vi "Backup.vi"() -> ()   [LabVIEW 2013]
uses:
  GUI_Template/GUI_master/tcp_new_data_event.ctl
  GUI_Template/GUI_master/tcp new data cluster.ctl
  <vilib>/vision/NI_Vision_Development_Module.lvlib
panel:
  out "MagSpec Lineout":cluster{"energy":dbl[], "counts":dbl[]}[](graph)=[{"energy"=array[427 elements], "counts"=[480.0, 481.0, 470.0, 482.0, 477.0, 480.0, 479.0, 479.0, 480.0, 485.0, 481.0, 484.0, 483.0, 482.0, 483.0, 477.0, 477.0, 475.0, 479.0, 479.0, 485.0, 477.0, 480.0, 478.0, 475.0, 485.0, 477.0, 485.0, 472.0, 479.0, 479.0, 472.0, 480.0, 481.0, 482.0, 481.0, 479.0, 477.0, 481.0, 486.0, 477.0, 477.0, 482.0, 481.0, 493.0, 474.0, 491.0, 486.0, 494.0, 488.0, 508.0, 495.0, 494.0, 499.0, 511.0, 500.0, 503.0, 501.0, 496.0, 499.0, 497.0, 500.0, 496.0, 503.0, 501.0, 504.0, 493.0, 492.0, 492.0, 492.0, 500.0, 494.0, 506.0, 494.0, 498.0, 492.0, 498.0, 503.0, 507.0, 498.0, 507.0, 504.0, 506.0, 504.0, 505.0, 503.0, 509.0, 501.0, 502.0, 500.0, 500.0, 496.0, 490.0, 491.0, 483.0, 490.0, 484.0, 469.0, 473.0, 469.0, 469.0, 469.0, 456.0, 465.0, 456.0, 458.0, 451.0, 445.0, 450.0, 443.0, 454.0, 438.0, 434.0, 440.0, 442.0, 450.0, 447.0, 447.0, 450.0, 446.0, 444.0, 446.0, 445.0, 433.0, 449.0, 444.0, 443.0, 441.0, 440.0, 436.0, 444.0, 440.0, 439.0, 435.0, 438.0, 430.0, 435.0, 432.0, 428.0, 433.0, 432.0, 430.0, 434.0, 428.0, 441.0, 426.0, 429.0, 427.0, 425.0, 423.0, 424.0, 419.0, 423.0, 428.0, 423.0, 423.0, 421.0, 423.0, 425.0, 425.0, 419.0, 426.0, 430.0, 429.0, 423.0, 423.0, 422.0, 421.0, 427.0, 426.0, 427.0, 420.0, 416.0, 428.0, 422.0, 420.0, 420.0, 422.0, 428.0, 423.0, 433.0, 417.0, 431.0, 419.0, 428.0, 427.0, 423.0, 417.0, 427.0, 419.0, 422.0, 421.0, 427.0, 420.0, 426.0, 419.0, 430.0, 422.0, 425.0, 426.0, 426.0, 422.0, 434.0, 427.0, 425.0, 430.0, 437.0, 434.0, 432.0, 441.0, 434.0, 435.0, 433.0, 434.0, 439.0, 434.0, 441.0, 436.0, 442.0, 440.0, 443.0, 446.0, 449.0, 441.0, 444.0, 441.0, 448.0, 455.0, 462.0, 450.0, 452.0, 452.0, 465.0, 463.0, 469.0, 466.0, 464.0, 462.0, 476.0, 460.0, 462.0, 475.0, 472.0, 473.0, 477.0, 471.0, 485.0, 474.0, 491.0, 482.0, 485.0, 492.0, 494.0, 498.0, 503.0, 491.0, 500.0, 501.0, 516.0, 500.0, 507.0, 515.0, 523.0, 517.0, 519.0, 525.0, 523.0, 521.0, 524.0, 528.0, 537.0, 533.0, 533.0, 542.0, 548.0, 538.0, 551.0, 563.0, 557.0, 565.0, 559.0, 570.0, 565.0, 580.0, 580.0, 578.0, 586.0, 591.0, 596.0, 605.0, 609.0, 607.0, 614.0, 620.0, 621.0, 628.0, 634.0, 642.0, 654.0, 646.0, 661.0, 654.0, 667.0, 676.0, 681.0, 683.0, 689.0, 703.0, 706.0, 725.0, 719.0, 744.0, 747.0, 757.0, 763.0, 773.0, 794.0, 795.0, 808.0, 821.0, 835.0, 838.0, 853.0, 861.0, 869.0, 886.0, 911.0, 903.0, 902.0, 916.0, 935.0, 925.0, 941.0, 959.0, 967.0, 966.0, 984.0, 976.0, 987.0, 1012.0, 1017.0, 1022.0, 1033.0, 1050.0, 1054.0, 1058.0, 1058.0, 1075.0, 1086.0, 1087.0, 1103.0, 1101.0, 1110.0, 1112.0, 1126.0, 1138.0, 1134.0, 1144.0, 1157.0, 1154.0, 1160.0, 1163.0, 1169.0, 1171.0, 1182.0, 1188.0, 1205.0, 1211.0, 1227.0, 1220.0, 1233.0, 1235.0, 1238.0, 1243.0, 1277.0, 1277.0, 1288.0, 1312.0, 1332.0, 1352.0, 1362.0, 1370.0, 1389.0, 1395.0, 1421.0, 1435.0, 1454.0, 1462.0, 1485.0, 1494.0, 1503.0, 1520.0, 1543.0, 1547.0, 1566.0, 1577.0, 1593.0, 1602.0, 1618.0, 1614.0, 1617.0, 1635.0, 1639.0, 1657.0, 1672.0, 1671.0, 1687.0, 1690.0, 1698.0, 1721.0, 1734.0, 1738.0, 1760.0, 1753.0, 1769.0, 1785.0, 1780.0, 1802.0, 1812.0, 1813.0, 1836.0, 1833.0, 1846.0, 1851.0, 1867.0, 1867.0, 1877.0]}, {"energy"=array[422 elements], "counts"=[1920.0, 1960.0, 1978.0, 1986.0, 2002.0, 2034.0, 2037.0, 2038.0, 2026.0, 2017.0, 2022.0, 2022.0, 2018.0, 2053.0, 2099.0, 2108.0, 2128.0, 2125.0, 2140.0, 2134.0, 2113.0, 2043.0, 1933.0, 1867.0, 1774.0, 1644.0, 1490.0, 1401.0, 1400.0, 1387.0, 1372.0, 1371.0, 1376.0, 1391.0, 1450.0, 1556.0, 1656.0, 1756.0, 1813.0, 1848.0, 1821.0, 1828.0, 1878.0, 1905.0, 1924.0, 1942.0, 1951.0, 1931.0, 1918.0, 1911.0, 1908.0, 1907.0, 1901.0, 1880.0, 1802.0, 1645.0, 1677.0, 1822.0, 1845.0, 1854.0, 1852.0, 1859.0, 1860.0, 1856.0, 1847.0, 1859.0, 1851.0, 1834.0, 1846.0, 1825.0, 1796.0, 1816.0, 1790.0, 1790.0, 1768.0, 1765.0, 1739.0, 1738.0, 1724.0, 1712.0, 1701.0, 1668.0, 1651.0, 1623.0, 1523.0, 1495.0, 1579.0, 1586.0, 1585.0, 1569.0, 1553.0, 1538.0, 1524.0, 1521.0, 1493.0, 1498.0, 1482.0, 1474.0, 1449.0, 1435.0, 1422.0, 1435.0, 1428.0, 1421.0, 1409.0, 1409.0, 1397.0, 1393.0, 1373.0, 1361.0, 1348.0, 1349.0, 1318.0, 1284.0, 1227.0, 1271.0, 1281.0, 1285.0, 1262.0, 1274.0, 1262.0, 1266.0, 1247.0, 1241.0, 1229.0, 1227.0, 1205.0, 1207.0, 1183.0, 1171.0, 1175.0, 1171.0, 1168.0, 1166.0, 1147.0, 1155.0, 1133.0, 1135.0, 1132.0, 1120.0, 1106.0, 1091.0, 1080.0, 1031.0, 1029.0, 1065.0, 1054.0, 1067.0, 1054.0, 1042.0, 1039.0, 1041.0, 1034.0, 1021.0, 1020.0, 999.0, 989.0, 983.0, 972.0, 978.0, 965.0, 960.0, 946.0, 951.0, 942.0, 938.0, 924.0, 917.0, 906.0, 908.0, 902.0, 881.0, 857.0, 842.0, 848.0, 858.0, 853.0, 855.0, 866.0, 849.0, 848.0, 837.0, 826.0, 812.0, 778.0, 726.0, 696.0, 683.0, 698.0, 694.0, 683.0, 681.0, 697.0, 698.0, 672.0, 668.0, 660.0, 667.0, 672.0, 686.0, 695.0, 701.0, 685.0, 685.0, 735.0, 763.0, 773.0, 792.0, 785.0, 791.0, 786.0, 792.0, 782.0, 780.0, 771.0, 777.0, 774.0, 761.0, 762.0, 769.0, 770.0, 767.0, 774.0, 765.0, 766.0, 761.0, 759.0, 762.0, 753.0, 752.0, 745.0, 739.0, 716.0, 710.0, 728.0, 749.0, 745.0, 747.0, 732.0, 751.0, 739.0, 744.0, 729.0, 734.0, 727.0, 723.0, 721.0, 719.0, 713.0, 716.0, 715.0, 716.0, 703.0, 721.0, 704.0, 708.0, 698.0, 695.0, 688.0, 692.0, 674.0, 678.0, 632.0, 646.0, 659.0, 679.0, 676.0, 674.0, 669.0, 664.0, 659.0, 668.0, 654.0, 650.0, 645.0, 650.0, 640.0, 635.0, 630.0, 635.0, 630.0, 637.0, 622.0, 621.0, 626.0, 614.0, 606.0, 614.0, 599.0, 597.0, 589.0, 580.0, 564.0, 575.0, 584.0, 590.0, 584.0, 585.0, 579.0, 582.0, 578.0, 571.0, 573.0, 574.0, 560.0, 559.0, 553.0, 547.0, 545.0, 554.0, 544.0, 553.0, 537.0, 540.0, 536.0, 539.0, 531.0, 525.0, 527.0, 522.0, 511.0, 497.0, 482.0, 503.0, 507.0, 515.0, 501.0, 503.0, 503.0, 502.0, 492.0, 485.0, 485.0, 483.0, 481.0, 479.0, 475.0, 460.0, 467.0, 462.0, 461.0, 466.0, 460.0, 463.0, 452.0, 448.0, 453.0, 446.0, 438.0, 423.0, 407.0, 366.0, 390.0, 423.0, 422.0, 433.0, 428.0, 418.0, 409.0, 419.0, 412.0, 418.0, 410.0, 407.0, 401.0, 397.0, 393.0, 404.0, 395.0, 390.0, 388.0, 395.0, 387.0, 386.0, 383.0, 385.0, 372.0, 370.0, 361.0, 360.0, 338.0, 338.0, 352.0, 364.0, 358.0, 351.0, 350.0, 348.0, 344.0, 346.0, 344.0, 343.0, 335.0, 340.0, 326.0, 327.0, 327.0, 328.0, 330.0, 328.0, 326.0, 316.0, 317.0, 320.0, 312.0, 325.0, 305.0, 306.0, 301.0, 287.0, 271.0, 290.0, 296.0, 294.0, 290.0, 293.0, 295.0, 284.0, 286.0, 283.0, 279.0, 281.0]}, {"energy"=array[479 elements], "counts"=array[479 elements]}]
  in  "confg cluster Cam2":T1={"position"=19.22, "field of view"=279.27, "Analysis ROI"=[23, 41, 501, 146]}
  in  "confg cluster Cam1":T1={"position"=142.68, "field of view"=174.3, "Analysis ROI"=[20, 85, 441, 119]}
  in  "confg cluster Cam0":T1={"position"=45.72, "field of view"=106.18, "Analysis ROI"=[50, 122, 476, 184]}
  out "image::5":T2(plugin-control) caption="MagSpec2"
  out "MagSpec2":u8[][](graph)
  out "error out":errorcluster
  out "image::4":T2(plugin-control) caption="MagSpec1"
  out "MagSpec1":u8[][](graph)
  in  "GUIdevice 5":string="10TW_MagSpec2"
  in  "GUIdevice 4":string="10TW_MagSpec1"
  out "MagSpec0":u8[][](graph)
  out "image::3":T2(plugin-control) caption="MagSpec0"
  in  "GUIdevice 3":string="10TW_MagSpec0"
  out "Status\n% - Ready":dbl(slide) scale=0.0..100.0
  out "AnalogOutput.Channel 0::1":dbl caption="Current Output" min=-10.0 max=10.0
  out "reading.var 5::2":dbl=-0.163229 caption="Current FeedBack" min=-100000.0 max=100000.0
  in  "GUIdevice 2":string="10TW_DAQmultiplier"
  in  "Magnet Current":dbl=-0.163229
  in  "GUIdevice 1":string="10TW_DAQ"
  in  "stop":bool
  out "tcp data event":T3
  out "error IO 2":errorcluster
  # "MAGNET CONTROLS"
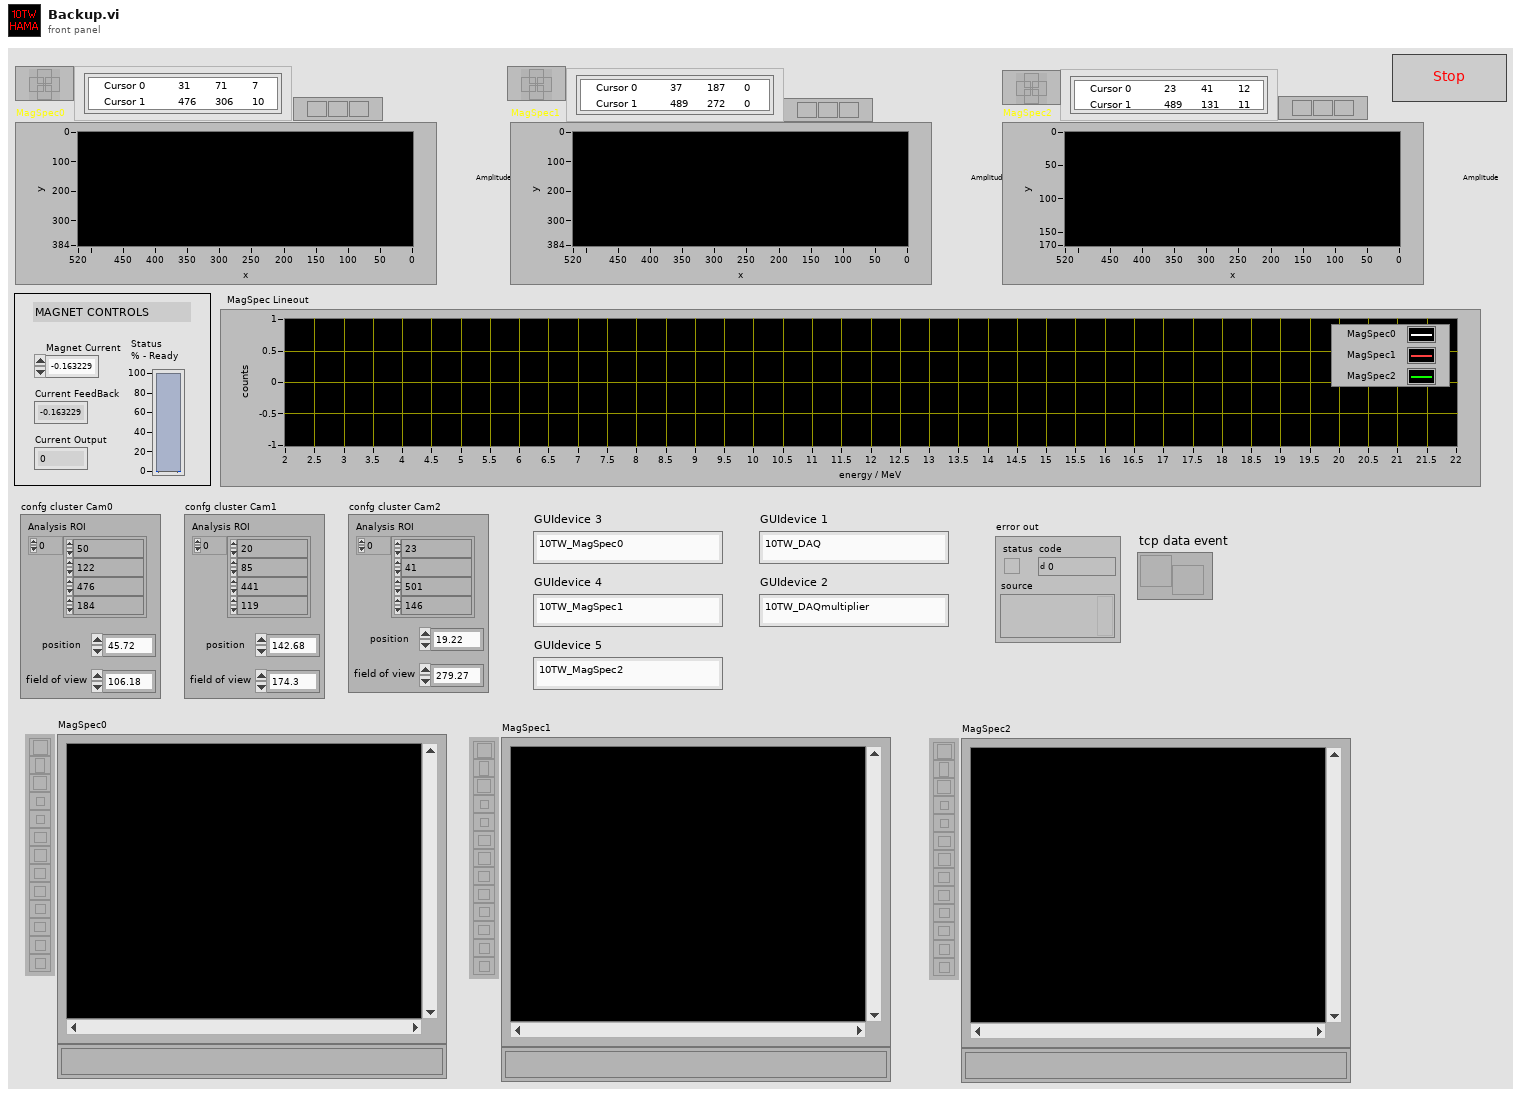
[diagram p1: front panel]
types:
  T1 = cluster{"position":dbl, "field of view":dbl, "Analysis ROI":i32[]}
  T2 = typedef "IMAQ Image.ctl" = refnum<image>
  T3 = typedef "tcp_new_data_event.ctl" = refnum<user-event>
  T4 = typedef "Image Type" = u32
  T5 = typedef "tcp new data cluster.ctl" = cluster{"EventEnum":enum16{"new data", "connection status update"}, "Device name":string}
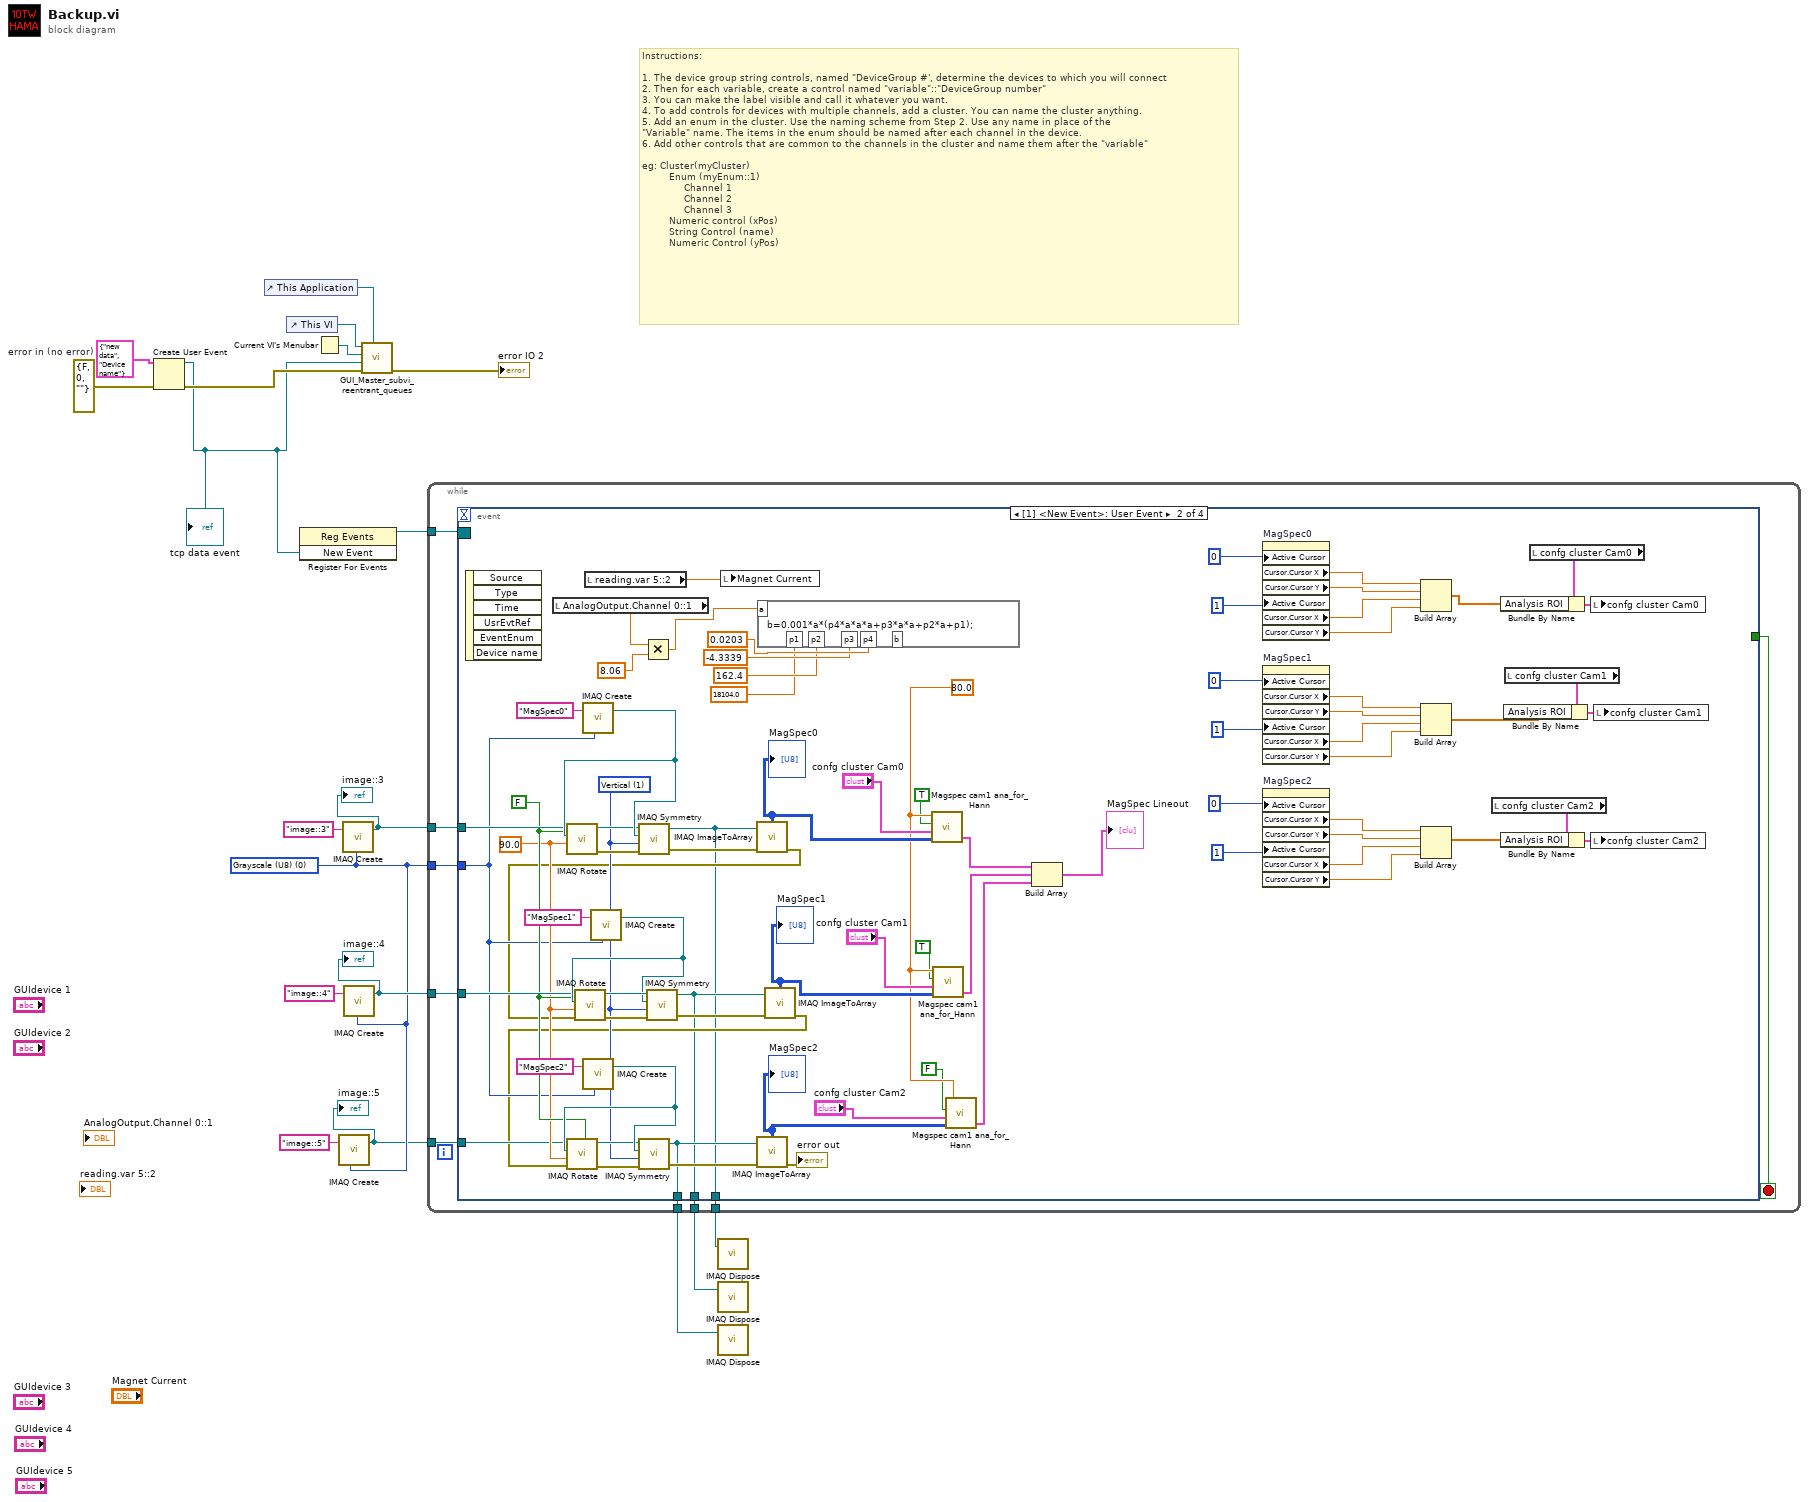
[diagram p0: block diagram]
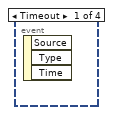
[diagram p2: hidden frame]
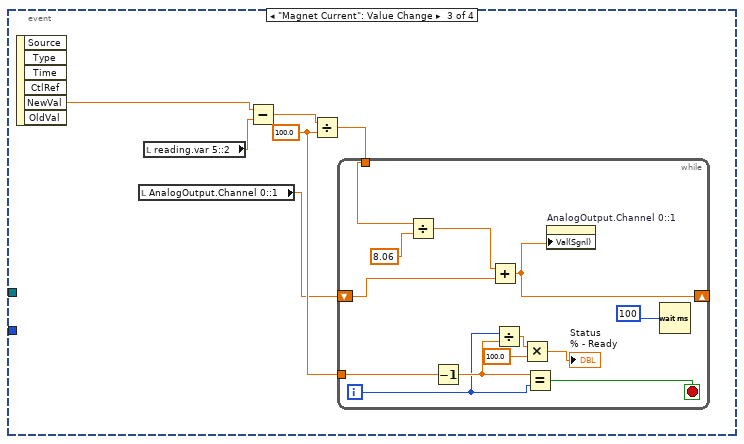
[diagram p3: hidden frame]
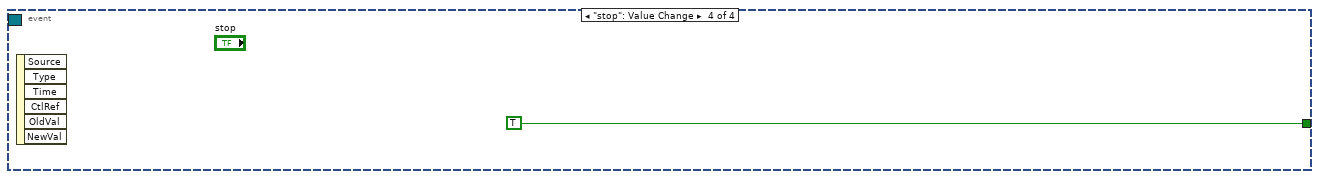
[diagram p4: hidden frame]
diagram:
  w5 = T4 0 items=["Grayscale (U8)", "Grayscale (I16)", "Grayscale (SGL)", "Complex (CSG)", "RGB (U32)", "HSL (U32)", "RGB (U64)", "Grayscale (U16)"] ("Image Type")
  w13 = errorcluster {"status"=FALSE, "code"=0, "source"=""}  # error in (no error)
  # "Instructions:\n\n1. The device group string controls, named \"DeviceGroup #', determine the devices to which you will connect\n2. Then for each variable, create a control named \"variable\"::\"DeviceGroup number\"\n3. You can make the label visible and call it whatever you want.\n4. To add controls for devices with multiple channels, add a cluster. You can name the cluster anything.\n5. Add an enum in the cluster. Use the naming scheme from Step 2. Use any name in place of the \n\"Variable\" name. The items in the enum should be named after each channel in the device. \n6. Add other controls that are common to the channels in the cluster and name them after the \"variable\"\n\neg: Cluster(myCluster)\n         Enum (myEnum::1)\n              Channel 1 \n              Channel 2\n              Channel 3\n         Numeric control (xPos)\n         String Control (name)\n         Numeric Control (yPos)"
  n1 = Create User Event(user event datatype=T5 {"EventEnum"=enum."new data", "Device name"="Device name"} ("New Event"), error in=w13) -> (user event=w12:refnum<user-event>, error out=w15:errorcluster)
  "tcp data event" <- w12
  n2 = control-ref of="This Application"() -> (w14:refnum<vi>)
  n3 = control-ref of="This VI"() -> (w18:refnum<vi>)
  n4 = register-events(w12) -> (reference out=w11:refnum<event-registration>)  [unwired: 2 in, 1 out]
  n5 = Current VI's Menubar() -> (w17:refnum<k9>)
  n6 = call "IMAQ Create"("Image Name"="image::5", "Image Type"=w5) -> ("New Image"=w4:T2)  [unwired: 3 in, 1 out]
  "image::5" <- w4
  n7 = call "IMAQ Create"("Image Name"="image::3", "Image Type"=w5) -> ("New Image"=w9:T2)  [unwired: 3 in, 1 out]
  "image::3" <- w9
  n8 = call "IMAQ Create"("Image Name"="image::4", "Image Type"=w5) -> ("New Image"=w7:T2)  [unwired: 3 in, 1 out]
  "image::4" <- w7
  n9 = call "GUI_Master_subvi_reentrant_queues.vi"("This Application"=w14, "error in (no error)"=w15, "tcp data event"=w12, "Caller menu reference"=w17, "Caller VI ref"=w18) -> ("error out"=→"error IO 2":errorcluster)  [unwired: 6 in]
  n10 = while {
    tunnel: w11 -> [w28]
    tunnel: w9 -> [w26]
    tunnel: w5 -> [w25]
    tunnel: w7 -> [w24]
    tunnel: w4 -> [w23]
    tunnel: [w22] -> w3
    tunnel: [w21] -> w2
    tunnel: [w20] -> w1
    stop <- w27 stop-if-true
    n11 = event shown="[1] <New Event>: User Event" {
      selector: w28 -> [_ _ _ _]
      dyn-events: _ -> [_ _ _ _]
      timeout: _ -> [_ _ _ _]
      tunnel: [_ _ _ TRUE] -> w27
      tunnel: w26 -> [_ w99 _ _]
      tunnel: w25 -> [_ w83 _ _]
      tunnel: w24 -> [_ w93 _ _]
      tunnel: w23 -> [_ w82 _ _]
      tunnel: [_ w79 _ _] -> w22
      tunnel: [_ w78 _ _] -> w21
      tunnel: [_ w77 _ _] -> w20
      event Timeout {
        n12 = event-data() -> ()  [unwired: 1 in, 3 out]
      }
      event User Event {
        w32 = 80.0 ("B [mT]")
        w86 = u32 1 items=["Horizontal", "Vertical", "Central", "1st Diagonal", "2nd Diagonal"] ("Type of Symmetry")
        w85 = FALSE ("Maintain Size")
        w84 = sgl 90.0 ("Angle (degrees)")
        n13 = event-data() -> ()  [unwired: 1 in, 6 out]
        n14 = local read "AnalogOutput.Channel 0::1"() -> (w72:dbl)
        n15 = call "IMAQ Create"("Image Name"="MagSpec0", "Image Type"=w83) -> ("New Image"=w103:T2)  [unwired: 3 in, 1 out]
        n16 = call "IMAQ Rotate"("Maintain Size"=w85, "Angle (degrees)"=w84, "Image Dst"=w103, "Image Src"=w99) -> ("error out"=w101:errorcluster, "Image Dst Out"=w100:T2)  [unwired: 4 in, 2 out]
        n17 = call "IMAQ Create"("Image Name"="MagSpec2", "Image Type"=w83) -> ("New Image"=w90:T2)  [unwired: 3 in, 1 out]
        n18 = local read "reading.var 5::2"() -> (w105:dbl)
        n19 = call "IMAQ Create"("Image Name"="MagSpec1", "Image Type"=w83) -> ("New Image"=w95:T2)  [unwired: 3 in, 1 out]
        n20 = call "IMAQ Symmetry"("error in (no error)"=w101, "Type of Symmetry"=w86, "Image Dst"=w103, "Image Src"=w100) -> ("error out"=w104:errorcluster, "Image Dst Out"=w77:T2)  [unwired: 1 out]
        n21 = Multiply(x=w72, y=8.06) -> (x*y=w70:dbl)
        n22 = local write "Magnet Current"(w105) -> ()
        n23 = call "IMAQ ImageToArray"("error in (no error)"=w104, "Image"=w77) -> ("error out"=w81:errorcluster, "Image Pixels (U8)"=w40:u8[][])  [unwired: 1 in, 4 out]
        "MagSpec0" <- w40
        n24 = call "IMAQ Rotate"("Maintain Size"=w85, "error in (no error)"=w81, "Angle (degrees)"=w84, "Image Dst"=w95, "Image Src"=w93) -> ("error out"=w97:errorcluster, "Image Dst Out"=w98:T2)  [unwired: 3 in, 2 out]
        n25 = call "IMAQ Symmetry"("error in (no error)"=w97, "Type of Symmetry"=w86, "Image Dst"=w95, "Image Src"=w98) -> ("error out"=w94:errorcluster, "Image Dst Out"=w78:T2)  [unwired: 1 out]
        n26 = formula code="b=0.001*a*(p4*a*a*a+p3*a*a+p2*a+p1);"("a"=w70, "p4"=0.0203 ("input variable"), "p3"=-4.3339 ("input variable"), "p2"=162.4 ("input variable"), "p1"=18104.0 ("input variable")) -> ()  [unwired: 1 out]
        n27 = call "IMAQ ImageToArray"("error in (no error)"=w94, "Image"=w78) -> ("error out"=w80:errorcluster, "Image Pixels (U8)"=w37:u8[][])  [unwired: 1 in, 4 out]
        "MagSpec1" <- w37
        n28 = call "IMAQ Rotate"("Maintain Size"=w85, "error in (no error)"=w80, "Angle (degrees)"=w84, "Image Dst"=w90, "Image Src"=w82) -> ("error out"=w88:errorcluster, "Image Dst Out"=w87:T2)  [unwired: 3 in, 2 out]
        n29 = call "IMAQ Symmetry"("error in (no error)"=w88, "Type of Symmetry"=w86, "Image Dst"=w90, "Image Src"=w87) -> ("error out"=w91:errorcluster, "Image Dst Out"=w79:T2)  [unwired: 1 out]
        n30 = call "IMAQ ImageToArray"("error in (no error)"=w91, "Image"=w79) -> ("error out"=→"error out":errorcluster, "Image Pixels (U8)"=w34:u8[][])  [unwired: 1 in, 4 out]
        "MagSpec2" <- w34
        n31 = call "Magspec cam1 ana_for_Hann.vi"("Image I16"=w40, "confg cluster"="confg cluster Cam0", "true4Fwd"=TRUE, "B [mT]"=w32) -> ("XY Graph"=w39:cluster{"energy":dbl[], "counts":dbl[]})  [unwired: 2 out]
        n32 = call "Magspec cam1 ana_for_Hann.vi"("Image I16"=w37, "confg cluster"="confg cluster Cam1", "true4Fwd"=TRUE, "B [mT]"=w32) -> ("XY Graph"=w36:cluster{"energy":dbl[], "counts":dbl[]})  [unwired: 2 out]
        n33 = call "Magspec cam1 ana_for_Hann.vi"("Image I16"=w34, "confg cluster"="confg cluster Cam2", "true4Fwd"=FALSE, "B [mT]"=w32) -> ("XY Graph"=w35:cluster{"energy":dbl[], "counts":dbl[]})  [unwired: 2 out]
        n34 = Build Array(w39, w36, w35) -> (→"MagSpec Lineout":cluster{"energy":dbl[], "counts":dbl[]}[])
        n35 = property on="MagSpec0" class="IntGraph (strict)"("Active Cursor"=u32 0, "Active Cursor"=u32 1) -> ("Cursor.Cursor X"=w66:dbl, "Cursor.Cursor Y"=w67:dbl, "Cursor.Cursor X"=w68:dbl, "Cursor.Cursor Y"=w63:dbl)  [unwired: 2 in, 2 out]
        n36 = property on="MagSpec1" class="IntGraph (strict)"("Active Cursor"=u32 0, "Active Cursor"=u32 1) -> ("Cursor.Cursor X"=w59:dbl, "Cursor.Cursor Y"=w58:dbl, "Cursor.Cursor X"=w57:dbl, "Cursor.Cursor Y"=w62:dbl)  [unwired: 2 in, 2 out]
        n37 = property on="MagSpec2" class="IntGraph (strict)"("Active Cursor"=u32 0, "Active Cursor"=u32 1) -> ("Cursor.Cursor X"=w54:dbl, "Cursor.Cursor Y"=w55:dbl, "Cursor.Cursor X"=w56:dbl, "Cursor.Cursor Y"=w51:dbl)  [unwired: 2 in, 2 out]
        n38 = Build Array(w66, w67, w68, w63) -> (w50:dbl[])
        n39 = Build Array(w59, w58, w57, w62) -> (w45:dbl[])
        n40 = Build Array(w54, w55, w56, w51) -> (w43:dbl[])
        n41 = local read "confg cluster Cam2"() -> (w44:T1)
        n42 = Bundle By Name(cluster=w44, "Analysis ROI"=w43) -> (w42:T1)
        n43 = local read "confg cluster Cam1"() -> (w47:T1)
        n44 = Bundle By Name(cluster=w47, "Analysis ROI"=w45) -> (w46:T1)
        n45 = local read "confg cluster Cam0"() -> (w49:T1)
        n46 = Bundle By Name(cluster=w49, "Analysis ROI"=w50) -> (w48:T1)
        n47 = local write "confg cluster Cam0"(w48) -> ()
        n48 = local write "confg cluster Cam2"(w42) -> ()
        n49 = local write "confg cluster Cam1"(w46) -> ()
      }
      event "Magnet Current": Value Change {
        w110 = 100.0 ("y")
        n50 = event-data() -> ("NewVal"=w107:dbl)  [unwired: 1 in, 5 out]
        n51 = local read "AnalogOutput.Channel 0::1"() -> (w106:dbl)
        n52 = local read "reading.var 5::2"() -> (w111:dbl)
        n53 = Subtract(x=w107, y=w111) -> (x-y=w109:dbl)
        n54 = Divide(x=w109, y=w110) -> (x/y=w108:dbl)
        n55 = while {
          tunnel: w110 -> [w122]
          tunnel: w108 -> [w116]
          shift-right: [w112] -> _
          shift-left: w106 -> [w113]
          i -> [w120]
          stop <- w124 stop-if-true
          n56 = Divide(x=w116, y=8.06) -> (x/y=w115:dbl)
          n57 = Decrement(x=w122) -> (x-1=w121:dbl)
          n58 = Add(x=w115, y=w113) -> (x+y=w112:dbl)
          n59 = Divide(x=w120, y=w121) -> (x/y=w119:dbl)
          n60 = Multiply(x=w119, y=100.0) -> (x*y=→"Status\n% - Ready":dbl)
          n61 = Equal?(x=w121, y=w120) -> (x = y?=w124:bool)
          n62 = property on="AnalogOutput.Channel 0::1" class="DigNum (strict)"("Val(Sgnl)"=w112) -> ()  [unwired: 2 in, 2 out]
          n63 = Wait (ms)(milliseconds to wait=u32 100) -> ()  [unwired: 1 out]
        }
      }
      event "stop": Value Change {
        n64 = event-data() -> ()  [unwired: 1 in, 6 out]
      }
    }
  }
  n65 = call "IMAQ Dispose"("Image"=w1) -> ()  [unwired: 5 in, 1 out]
  n66 = call "IMAQ Dispose"("Image"=w2) -> ()  [unwired: 5 in, 1 out]
  n67 = call "IMAQ Dispose"("Image"=w3) -> ()  [unwired: 5 in, 1 out]
